vi "Main_2018.vi"() -> ()   [LabVIEW 2013]
uses:
  Proyecto/Test_Libraries.lvlib
  <vilib>/Utility/NIReport.llb/NI_report.lvclass
  Selector.ctl
  <vilib>/Utility/NIReport.llb/Report Type.ctl
  <vilib>/Utility/NIReport.llb/NI_ReportGenerationCore.lvlib
panel:
  out "Refresh time (s)":dbl
  in  "Number of samples":i32=50
  in  "Rate (Hz)":dbl=100.0
  out "Path":bool
  out "RPM":bool
  out "Voltmeter":bool
  out "ACS712":bool
  out "Error DAQ":errorcluster[](array[cluster])
  out "Error path":errorcluster caption="error out"
  in  "Data Acquisition":bool
  in  "File Path":path
  in  "Time":i32=60
  out "Iteration":i32
  out "Timing loop (ms)":u32
  in  "Main":enum32{"Voltage", "Current", "RPM", "About"}(tab)
  out "Voltage":dbl(graph)
  out "Current":dbl(graph)
  out "Velocity":dbl(graph)
  in  "Stop":bool
  out "Current [A]":dbl(knob) scale=0.0..10.0 scale format="%#_3g"
  out "Voltage [V]":dbl(knob) scale=0.0..10.0
  out "Power [W]":dbl(knob) scale=0.0..500.0
  out "Velocity [RPM]":dbl(knob) scale=0.0..1800.0
  # "TEST BENCH FOR WIND TURBINE"
  # "Status & Error"
  # "DAQ Settings"
  # "Save data"
  # "Instituto Tecnológico de Costa Rica"
  # "Laboratorio de Investigación en Energía Eólica"
  # "Developer: B.S. Student. Brandon Obregón Garita"
  # "Email: bobregon@estudiantec.cr"
  # "Version: 1.0"
  # "Last modification: 28/08/2023"
  # "Optocoupler channel: Digital sensor, operational voltage: 5 [V].\n\nOut connected to PFI 0. GND connected to D.GND. \nVCC required 5 V of  external device [DC Power Supply]"
  # "Common ground for analog sensors"
  # "Current Channel [ACS712 - 30A]: Sensor required 5V of an external device. \nSensibility [based on Lab Test]: 0.070 mV/A\nOut connected to AI 0. GND connected to common ground\nMax Current: 30 A."
  # "Voltage Channel: Measured from voltage divider, protected by Zener Diode. Max Volt: 4.7 [V]\nPositive connected to AI 1 | Negative connected to common ground\nVoltage divider: 10kOhm & 1kOhm | Gain: Vturbine = 11*Vmeasured"
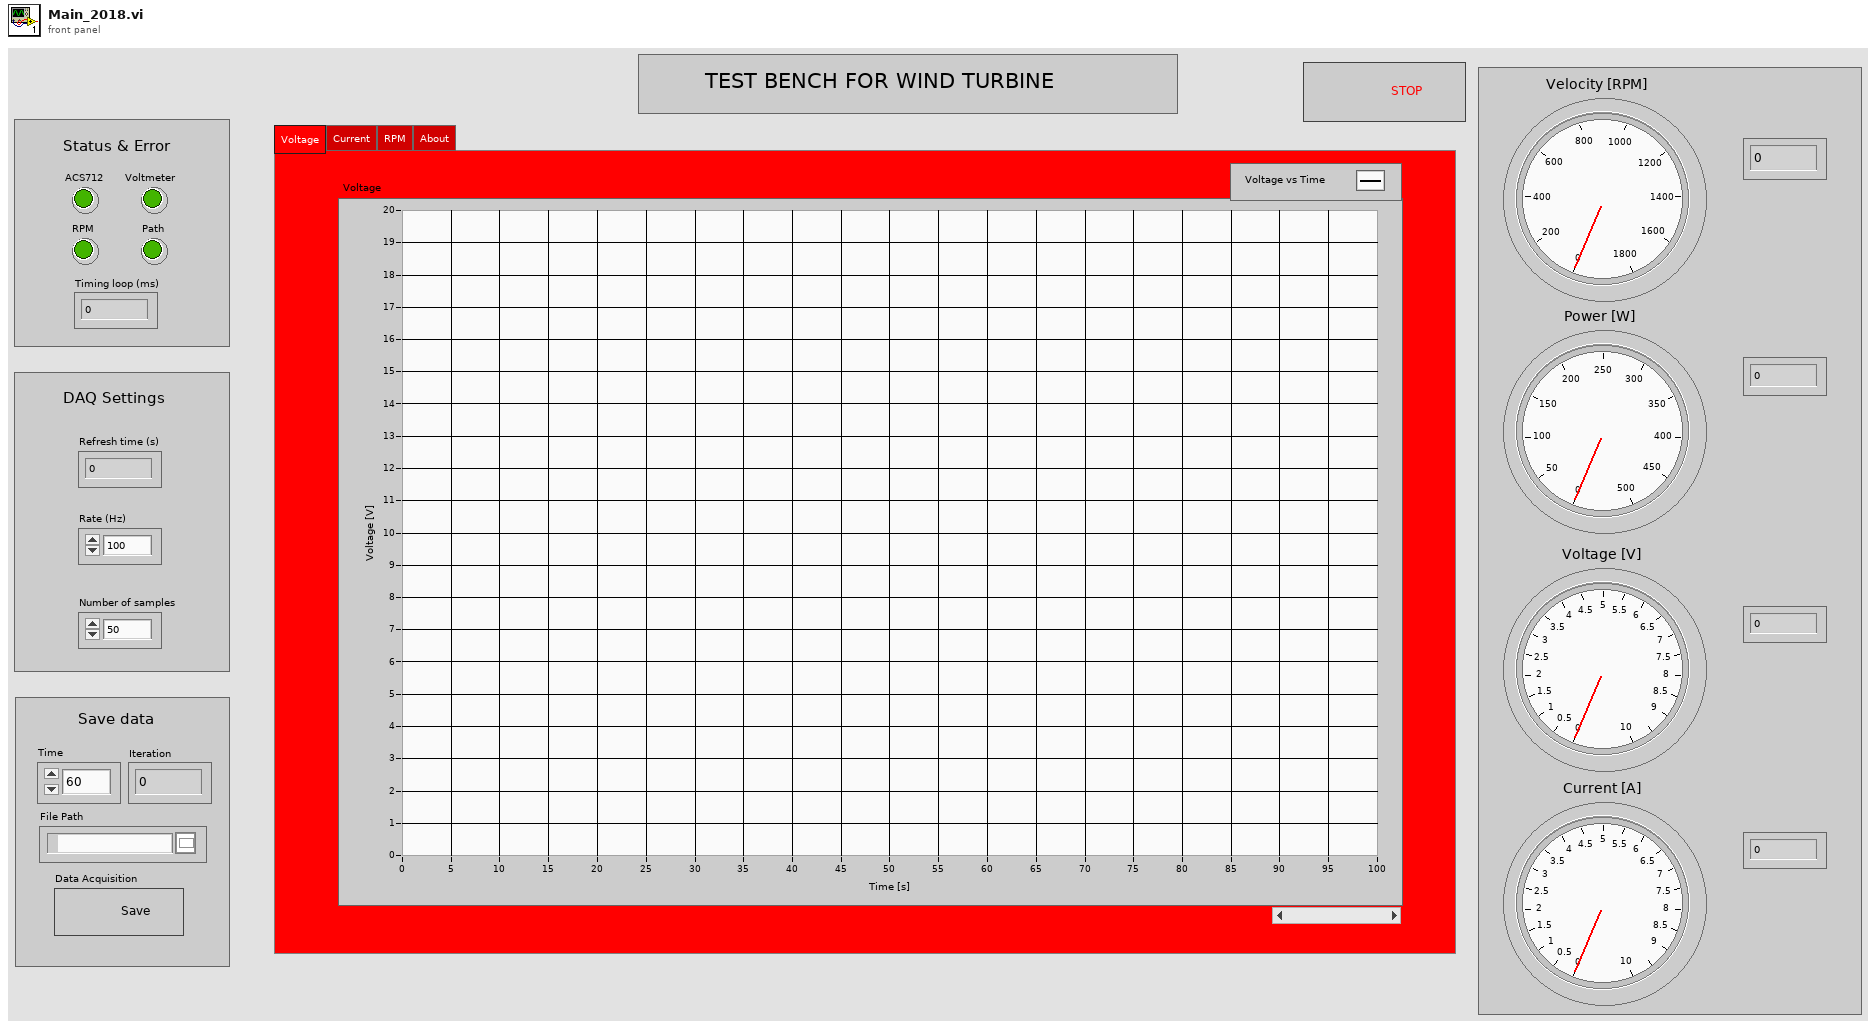
[diagram p1: front panel]
types:
  T1 = enum16{"maximized", "minimized", "normal", "no change"}
  T2 = typedef "NI_ReportGenerationCore.lvlib/Report Type.ctl" = enum16{"HTML", "Word", "Excel"}
  T3 = typedef "Test_Libraries.lvlib/Selector.ctl" = enum16{"Stand By", "Path", "Measurement", "End"}
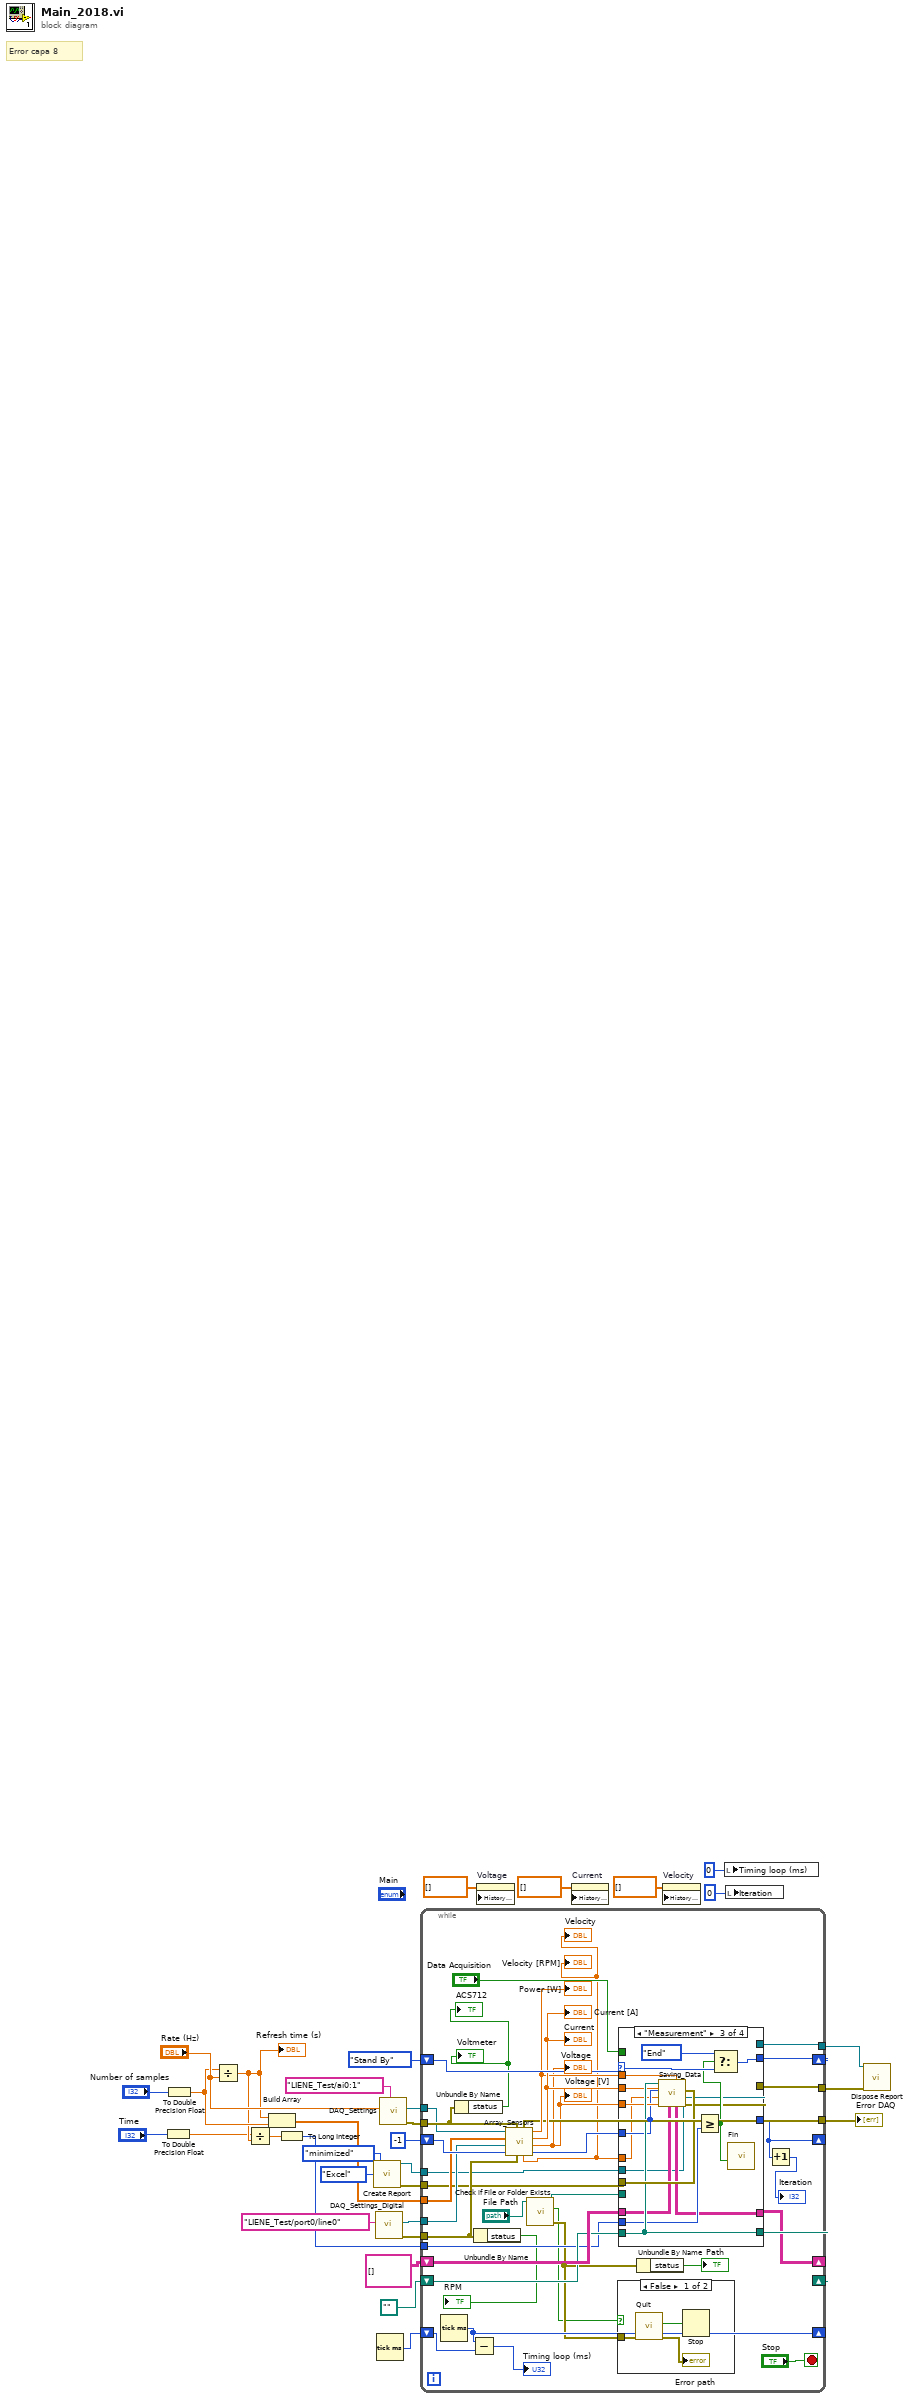
[diagram p0: block diagram]
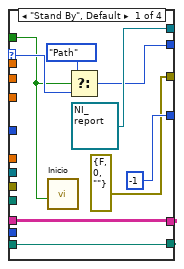
[diagram p3: hidden frame]
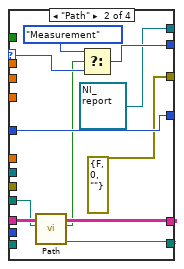
[diagram p4: hidden frame]
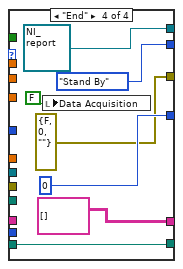
[diagram p5: hidden frame]
diagram:
  # "Error capa 8"
  n1 = To Double Precision Float(number="Time") -> (double precision float=w4:dbl)
  n2 = To Double Precision Float(number="Number of samples") -> (double precision float=w7:dbl)
  n3 = Divide(x=w7, y="Rate (Hz)") -> (x/y=w6:dbl)
  "Refresh time (s)" <- w6
  n4 = Divide(x=w4, y=w6) -> (x/y=w3:dbl)
  n5 = Build Array(w6, w7) -> (w9:dbl[])
  n6 = To Long Integer(number=w3) -> (32bit integer=w2:i32)
  n7 = call <vilib>:"Create Report.vi"("window state (normal)"=T1."minimized", "report type"=Report_Type."Excel") -> ("report out"=w12:refnum<class "NI_report.lvclass">, "error out"=w11:errorcluster)  [unwired: 12 in]
  n8 = call "DAQ_Settings_Digital.vi"("lines"=tag "LIENE_Test/port0/line0") -> ("error out"=w19:errorcluster, "task out"=w27:refnum<k21>)  [unwired: 9 in]
  n9 = Tick Count (ms)() -> (millisecond timer value=w23:u32)
  n10 = call "DAQ_Settings.vi"("Channel"=tag "LIENE_Test/ai0:1" ("physical channels"), "rate"="Rate (Hz)") -> ("error out"=w32:errorcluster, "task out"=w30:refnum<k21>)  [unwired: 8 in]
  n11 = while {
    tunnel: w30 -> [w58]
    tunnel: w27 -> [w57]
    shift-right: [w55] -> _
    shift-left: Selector."Stand By" ("Enum") -> [w66]
    shift-right: [w34] -> _
    shift-left: -1 -> [w68]
    tunnel: w2 -> [w53]
    shift-right: [w52] -> _
    shift-left: path "" ("appended path") -> [w59]
    shift-right: [w51] -> _
    shift-left: w23 -> [w50]
    tunnel: w32 -> [w62]
    tunnel: w19 -> [w61]
    tunnel: [w60] -> w18
    shift-right: [w42] -> _
    shift-left: string[][] [] ("Input") -> [w69]
    tunnel: [w38] -> w15
    tunnel: [w37] -> w14
    tunnel: w12 -> [w36]
    tunnel: w11 -> [w35]
    tunnel: w9 -> [w67]
    stop <- "Stop" stop-if-true
    n12 = Tick Count (ms)() -> (millisecond timer value=w51:u32)
    n13 = Unbundle By Name(w62) -> ("status"=→"ACS712" →"Voltmeter":bool)
    n14 = Subtract(x=w51, y=w50) -> (x-y=→"Timing loop (ms)":u32)
    n15 = Unbundle By Name(w61) -> ("status"=→"RPM":bool)
    n16 = call "Array_Sensors.vi"("error in 2"=w61, "error in"=w62, "Count"=w68, "Digital"=w57, "Array"=w67, "Analog"=w58) -> ("Iteración"=w56:i32, "Voltage_in"=w47:dbl, "Current"=w65:dbl, "Watt"=w64:dbl, "RPM"=w46:dbl, "appended array"=w60:errorcluster[])
    "Voltage" <- w47
    "Velocity [RPM]" <- w46
    "Power [W]" <- w64
    "Current [A]" <- w65
    "Voltage [V]" <- w47
    "Current" <- w65
    "Velocity" <- w46
    n17 = call <vilib>:"Check if File or Folder Exists.vi"("path"="File Path") -> ("error out"=w41:errorcluster, "file or folder exists?"=w40:bool, "dup path"=w63:path)  [unwired: 8 in]
    n18 = case shown="False" w40 {
      tunnel: w41 -> [w70 _]
      frame False {
        n19 = call "Quit"("error in (no error)"=w70) -> ("error out"=→"Error path":errorcluster, "OK"=w71:bool)  [unwired: 9 in]
        n20 = Stop(stop? (T)=w71) -> ()
      }
      frame True {
      }
    }
    n21 = case shown="\"Measurement\"" w66 {
      selector: w66 -> [w78 w86 w106 _]
      tunnel: w64 -> [_ _ w102 _]
      tunnel: w65 -> [_ _ w101 _]
      tunnel: w47 -> [_ _ w100 _]
      tunnel: w46 -> [_ _ w98 _]
      tunnel: w56 -> [_ w91 w99 _]
      tunnel: [-1 ("Count+1") w91 w99 0 ("Iteración")] -> w34
      tunnel: "Data Acquisition" -> [w75 _ _ _]
      tunnel: [w77 w88 w104 Selector."Stand By" ("Enum")] -> w55
      tunnel: w53 -> [_ _ w97 _]
      tunnel: [w76 w90 w107 w113] -> w52
      tunnel: w59 -> [w76 _ w107 w113]
      tunnel: w63 -> [_ w84 _ _]
      tunnel: w69 -> [w74 w87 w96 _]
      tunnel: [w74 w87 w95 string[][] [] ("output")] -> w42
      tunnel: w36 -> [_ _ w94 _]
      tunnel: w35 -> [_ _ w108 _]
      tunnel: [refnum<class "NI_report.lvclass"> refnum ("report out") refnum<class "NI_report.lvclass"> refnum ("report out") w93 refnum<class "NI_report.lvclass"> refnum ("report out")] -> w38
      tunnel: [errorcluster {"status"=FALSE, "code"=0, "source"=""} ("error out") errorcluster {"status"=FALSE, "code"=0, "source"=""} ("error out") w92 errorcluster {"status"=FALSE, "code"=0, "source"=""} ("error out")] -> w37
      frame "Stand By", Default {
        n22 = call "Inicio"("Enable"=w75) -> ()  [unwired: 9 in, 2 out]
        n23 = Select(t=Selector."Path" ("Enum"), s=w75, f=w78) -> (s? t:f=w77:T3)
      }
      frame "Path" {
        n24 = call "Path.vi"("selected path"=w84) -> ("appended path"=w90:path, "Boolean"=w85:bool)  [unwired: 7 in, 2 out]
        n25 = Select(t=Selector."Measurement" ("Enum"), s=w85, f=w86) -> (s? t:f=w88:T3)
      }
      frame "Measurement" {
        n26 = call "Saving_Data.vi"("error in"=w108, "report in"=w94, "Current"=w102, "Input"=w96, "Watt"=w101, "Voltage"=w100, "RPM"=w98, "Iteration"=w99, "Path"=w107) -> ("error out"=w92:errorcluster, "report out"=w93:refnum<class "NI_report.lvclass">, "output"=w95:string[][])
        n27 = Greater Or Equal?(x=w99, y=w97) -> (x >= y?=w103:bool)
        n28 = Select(t=Selector."End" ("Enum"), s=w103, f=w106) -> (s? t:f=w104:T3)
        n29 = call "Fin"("Enable"=w103) -> ()  [unwired: 9 in, 2 out]
      }
      frame "End" {
        n30 = local write "Data Acquisition"(FALSE ("Toma de datos")) -> ()
      }
    }
    n31 = Unbundle By Name(w41) -> ("status"=→"Path":bool)
    n32 = Increment(x=w34) -> (x+1=→"Iteration":i32)
  }
  "Error DAQ" <- w18
  n33 = property on="Voltage" class="WFChart (strict)"("History Data"=dbl[] []) -> ()  [unwired: 2 in, 2 out]
  n34 = property on="Current" class="WFChart (strict)"("History Data"=dbl[] []) -> ()  [unwired: 2 in, 2 out]
  n35 = property on="Velocity" class="WFChart (strict)"("History Data"=dbl[] []) -> ()  [unwired: 2 in, 2 out]
  n36 = local write "Timing loop (ms)"(u32 0 ("Loop time")) -> ()
  n37 = local write "Iteration"(0 ("Iteración")) -> ()
  n38 = call-dynamic "Dispose Report.vi"("report in"=w15, "error in (no error)"=w14) -> ()  [unwired: 13 in, 1 out]
